vi "set_error_color_test.vi"(6 "value_ref":refnum<vi>, 7 "value":dbl, 8 "lolo":dbl=-1e+100, 9 "lo":dbl=-1e+100, 10 "hi":dbl=1e+100, 11 "hihi":dbl=1e+100) -> ()   [LabVIEW 2019]
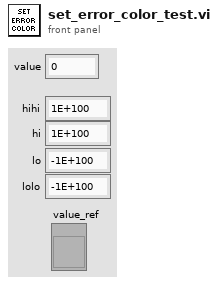
[diagram p1: front panel]
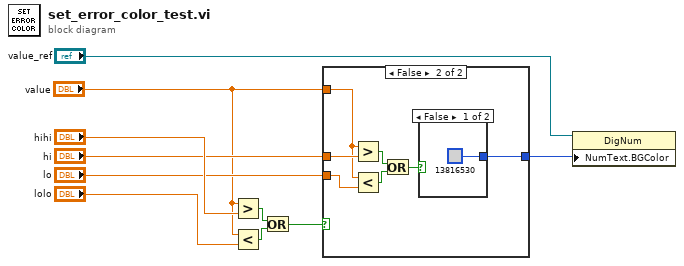
[diagram p0: block diagram]
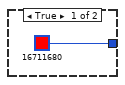
[diagram p2: hidden frame]
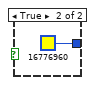
[diagram p3: hidden frame]
diagram:
  n1 = Greater?(x="value", y="hihi") -> (0:w6:bool)
  n2 = Less?(x="value", y="lolo") -> (x < y?=w5:bool)
  n3 = Or(x=w6, y=w5) -> (x .or. y?=w9:bool)
  n4 = case shown="False" w9 {
    tunnel: "hi" -> [_ w18]
    tunnel: "lo" -> [_ w17]
    tunnel: [u32 16711680 ("Numeric Text.Text Colors:BG Color") w13] -> w10
    tunnel: "value" -> [_ w12]
    frame True {
    }
    frame False {
      n5 = Greater?(x=w12, y=w18) -> (0:w15:bool)
      n6 = Less?(x=w12, y=w17) -> (x < y?=w16:bool)
      n7 = Or(x=w15, y=w16) -> (x .or. y?=w14:bool)
      n8 = case shown="False" w14 {
        tunnel: [u32 13816530 ("Numeric Text.Text Colors:BG Color") u32 16776960 ("Numeric Text.Text Colors:BG Color")] -> w13
        frame False {
        }
        frame True {
        }
      }
    }
  }
  n9 = property on="Property Node" class="DigNum"(reference="value_ref", "NumText.BGColor"=w10) -> ()  [unwired: 1 in, 2 out]
